vi "DzSysRem_ErrorCodes&Descs.vi"() -> (0 "AV_ErrorsDescs_Trans":cluster{"Code":i32, "Description":string}[](array[cluster])=[{"Code"=15001, "Description"="Timeout occured while waiting for the Dazzler to treat the request.\nPlease check the Dazzler software is in \"remote enable\" state."}] caption="Error Descriptions")   [LabVIEW 2012]
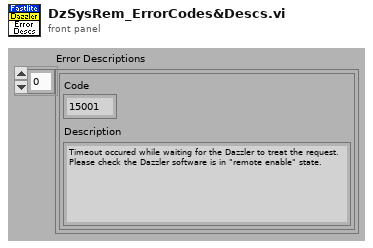
[diagram p1: front panel]
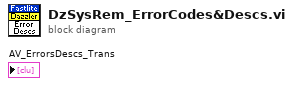
[diagram p0: block diagram]
diagram:
